vi "动态时值缓存指数压缩.vi"(6 "新数据":cluster{"时间":timestamp, "数值":dbl}, 11 "缓存数据":T1) -> (3 "缓存数据 o":T1)   [LabVIEW 2017, in "时值缓存压缩模块.lvlib"]
doc: "注意：\n缓存容量要在输入数据中设好，默认容量 300 点。"
panel:
  out "Error Out":errorcluster caption="错误输出"
  in  "Error In":errorcluster caption="错误输入"
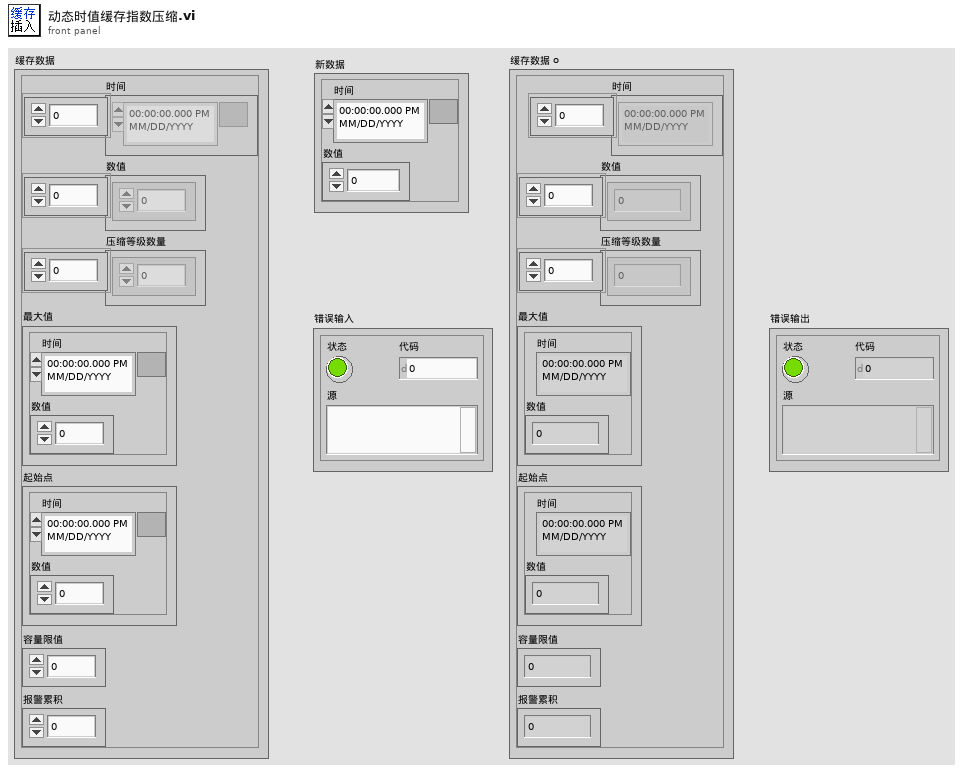
[diagram p1: front panel]
types:
  T1 = typedef "时值缓存压缩模块.lvlib/缓存数据.ctl" = cluster{"时间":timestamp[], "数值":dbl[], "压缩等级数量":i32[], "最大值":cluster{"时间":timestamp, "数值":dbl}, "起始点":cluster{"时间":timestamp, "数值":dbl}, "容量限值":i32, "报警累积":dbl}
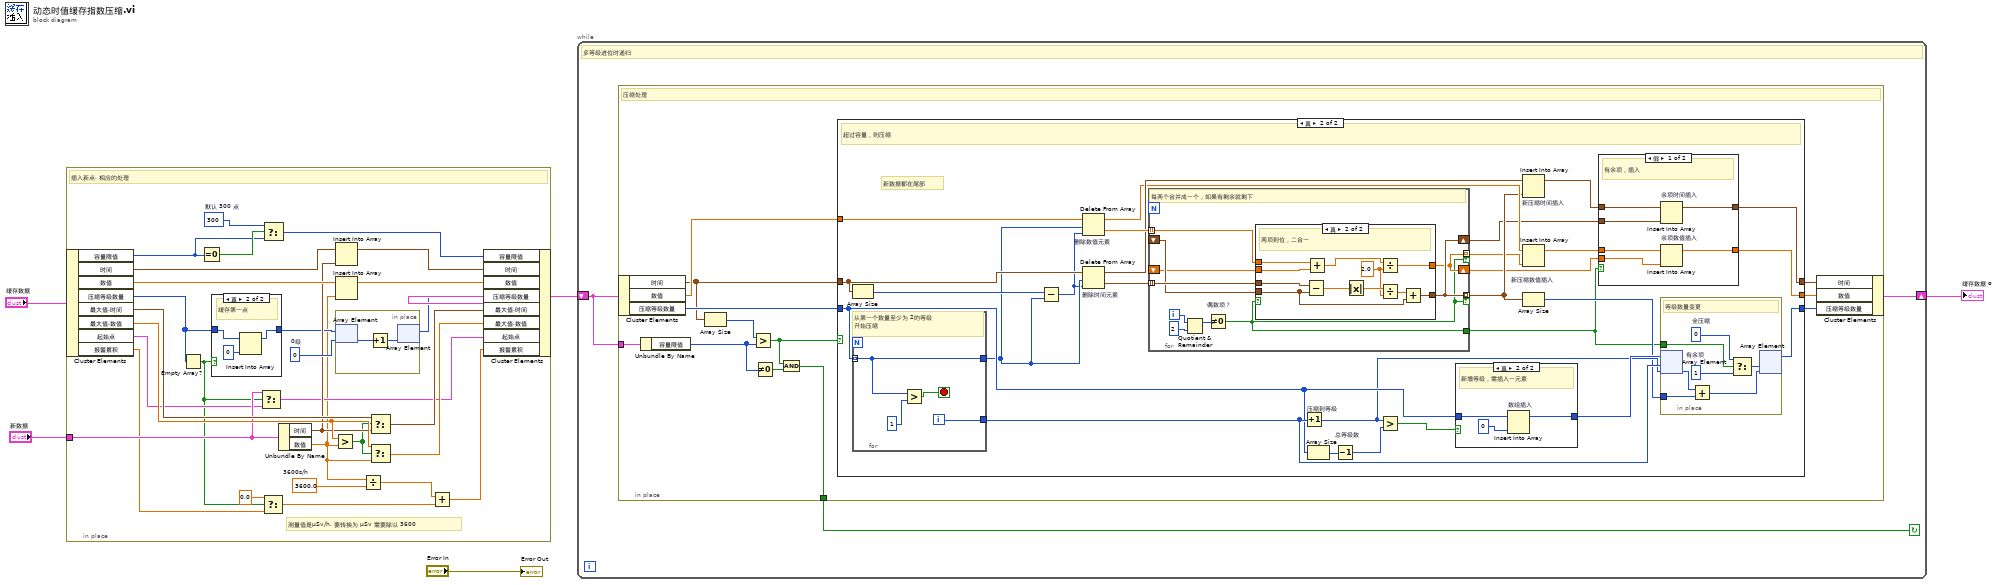
[diagram p0: block diagram]
diagram:
  n1 = in-place {
    in-place-border: "新数据" -> [w20]
    w6 = 3600.0  # 3600s/h
    w16 = 300  # 默认 300 点
    w32 = 0  # 0级
    # "测量值是μSv/h, 要转换为 μSv 需要除以 3600"
    # "插入新点, 相应的处理"
    n2 = in-place-cluster #1("缓存数据") -> ("容量限值"=w15:i32, "时间"=w34:timestamp[], "数值"=w33:dbl[], "压缩等级数量"=w22:i32[], "最大值.时间"=w28:timestamp, "最大值.数值"=w27:dbl, "起始点"=w19:cluster{"时间":timestamp, "数值":dbl}, "报警累积"=w10:dbl)
    n3 = Empty Array?(array=w22) -> (empty?=w12:bool)
    n4 = Equal To 0?(x=w15) -> (x = 0?=w17:bool)
    n5 = case shown="真" w12 {
      tunnel: w22 -> [w35 w38]
      tunnel: [w35 w36] -> w21
      frame False {
        # "不是第一点"
      }
      frame True {
        # "缓存第一点"
        n6 = Insert Into Array(array=w38, new element=0 ("新元素/子数组")) -> (w36:i32[])  [unwired: 1 in]
      }
    }
    n7 = Select(t=w20, s=w12, f=w19) -> (s? t:f=w18:cluster{"时间":timestamp, "数值":dbl})
    n8 = Select(t=0.0, s=w12, f=w10) -> (s? t:f=w9:dbl)
    n9 = Select(t=w16, s=w17, f=w15) -> (s? t:f=w14:i32)
    n10 = Unbundle By Name(w20) -> ("时间"=w26:timestamp, "数值"=w13:dbl)
    n11 = Greater?(x=w27, y=w13) -> (0:w25:bool)
    n12 = Insert Into Array(array=w34, new element=w26) -> (w29:timestamp[])  [unwired: 1 in]
    n13 = Insert Into Array(array=w33, new element=w13) -> (w30:dbl[])  [unwired: 1 in]
    n14 = in-place {
      n15 = in-place-array #2(w21, w32) -> (w40:i32)
      n16 = Increment(x=w40) -> (x+1=w39:i32)
      n17 = in-place-array #2(w39) -> (w31:i32[])  [unwired: 1 out]
    }
    n18 = Divide(x=w13, y=w6) -> (x/y=w7:dbl)
    n19 = Select(t=w28, s=w25, f=w26) -> (s? t:f=w24:timestamp)
    n20 = Select(t=w27, s=w25, f=w13) -> (s? t:f=w23:dbl)
    n21 = Add(x=w7, y=w9) -> (x+y=w8:dbl)
    n22 = in-place-cluster #1("容量限值"=w14, "时间"=w29, "数值"=w30, "压缩等级数量"=w31, "最大值.时间"=w24, "最大值.数值"=w23, "起始点"=w18, "报警累积"=w8) -> (w3:T1)
  }
  n23 = while {
    shift-right: [w42] -> w2
    shift-left: w3 -> [w43]
    stop <- w41 continue-if-true
    # "多等级进位时递归"
    n24 = in-place {
      in-place-border: w43 -> [w48]
      in-place-border: [w45] -> w41
      # "压缩处理"
      n25 = in-place-cluster #3(w43) -> ("时间"=w52:timestamp[], "数值"=w55:dbl[], "压缩等级数量"=w54:i32[])
      n26 = Unbundle By Name(w48) -> ("容量限值"=w46:i32)
      n27 = Array Size(array=w52) -> (size(s)=w53:i32)
      n28 = Greater?(x=w53, y=w46) -> (0:w47:bool)
      n29 = Not Equal To 0?(x=w46) -> (x != 0?=w44:bool)
      n30 = And(x=w47, y=w44) -> (x .and. y?=w45:bool)
      n31 = case shown="真" w47 {
        tunnel: w55 -> [w57 w73]
        tunnel: w52 -> [w58 w74]
        tunnel: [w58 w61] -> w51
        tunnel: [w57 w60] -> w50
        tunnel: [w56 w76] -> w49
        tunnel: w54 -> [w56 w80]
        frame False {
          # "没超过容量就通过"
        }
        frame True {
          # "新数据都在尾部"
          # "超过容量，则压缩"
          n32 = Array Size(array=w74) -> (size(s)=w85:i32)
          n33 = for {
            tunnel: w80 -> [w130] mode=indexing
            tunnel: [w131] -> w83
            tunnel: [w130] -> w72
            i -> [w131]
            stop <- w128 stop-if-true
            # "从第一个数量至少为 2的等级\n开始压缩"
            n34 = Greater?(x=w130, y=1) -> (0:w128:bool)
          }
          n35 = Subtract(x=w85, y=w72) -> (x-y=w71:i32)
          n36 = Delete From Array "删除数值元素"(array=w73, length=w72, index=w71) -> (deleted portion=w70:dbl[], array with subset deleted=w68:dbl[])
          n37 = Delete From Array "删除时间元素"(array=w74, length=w72, index=w71) -> (deleted portion=w75:timestamp[], array with subset deleted=w69:timestamp[])
          n38 = for {
            tunnel: w75 -> [w111] mode=indexing
            tunnel: w70 -> [w110] mode=indexing
            shift-right: [w107] -> w63
            shift-left: _ -> [w109]
            shift-right: [w106] -> w62
            shift-left: _ -> [w108]
            tunnel: [w107] -> w67 mode=indexing if=w105
            tunnel: [w106] -> w66 mode=indexing if=w105
            tunnel: [w105] -> w59
            i -> [w114]
            # "每两个合并成一个，如果有剩余就剩下"
            n39 = Quotient & Remainder(x=w114, y=2) -> (x-y*floor(x/y)=w112:i32)  [unwired: 1 out]
            n40 = Not Equal To 0? "偶数项？"(x=w112) -> (x != 0?=w105:bool)
            n41 = case shown="真" w105 {
              tunnel: [w116 w122] -> w107
              tunnel: w111 -> [w116 w127]
              tunnel: [w115 w118] -> w106
              tunnel: w110 -> [w115 w121]
              tunnel: w109 -> [_ w123]
              tunnel: w108 -> [_ w120]
              frame False {
                # "单独一项，传到下一帧"
              }
              frame True {
                w117 = 2.0 ("y")
                # "两项到位，二合一"
                n42 = Subtract(x=w127, y=w123) -> (x-y=w126:dbl)
                n43 = Add(x=w121, y=w120) -> (x+y=w119:dbl)
                n44 = Absolute Value(x=w126) -> (abs(x)=w125:dbl)
                n45 = Divide(x=w119, y=w117) -> (x/y=w118:dbl)
                n46 = Divide(x=w125, y=w117) -> (x/y=w124:dbl)
                n47 = Add(x=w124, y=w123) -> (x+y=w122:timestamp)
              }
            }
          }
          n48 = Increment "压缩到等级"(x=w83) -> (x+1=w78:i32)
          n49 = Array Size(array=w80) -> (size(s)=w84:i32)
          n50 = Decrement "总等级数"(x=w84) -> (x-1=w82:i32)
          n51 = Greater?(x=w78, y=w82) -> (0:w81:bool)
          n52 = case shown="真" w81 {
            tunnel: w80 -> [w94 w97]
            tunnel: [w94 w95] -> w79
            frame False {
              # "未新增等级，则通过"
            }
            frame True {
              # "新增等级，需插入一元素"
              n53 = Insert Into Array "数组插入"(array=w97, new element=0 ("新元素/子数组")) -> (w95:i32[])  [unwired: 1 in]
            }
          }
          n54 = Insert Into Array "新压缩时间插入"(array=w69, new element=w67) -> (w65:timestamp[])  [unwired: 1 in]
          n55 = Insert Into Array "新压缩数值插入"(array=w68, new element=w66) -> (w64:dbl[])  [unwired: 1 in]
          n56 = Array Size(array=w67) -> (size(s)=w77:i32)
          n57 = case shown="假" w59 {
            tunnel: w65 -> [w91 w93]
            tunnel: w64 -> [w90 w92]
            tunnel: w63 -> [w89 _]
            tunnel: w62 -> [w88 _]
            tunnel: [w87 w92] -> w60
            tunnel: [w86 w93] -> w61
            frame False {
              # "有余项，插入"
              n58 = Insert Into Array "余项时间插入"(array=w91, new element=w89) -> (w86:timestamp[])  [unwired: 1 in]
              n59 = Insert Into Array "余项数值插入"(array=w90, new element=w88) -> (w87:dbl[])  [unwired: 1 in]
            }
            frame True {
              # "全压缩，通过"
            }
          }
          n60 = in-place {
            in-place-border: w59 -> [w103]
            in-place-border: w77 -> [w98]
            w102 = 1  # 有余项
            w104 = 0  # 全压缩
            # "等级数量变更"
            n61 = in-place-array #4(w79, w83, w78) -> (w101:i32)  [unwired: 1 out]
            n62 = Add(x=w101, y=w98) -> (x+y=w99:i32)
            n63 = Select(t=w104, s=w103, f=w102) -> (s? t:f=w100:i32)
            n64 = in-place-array #4(w100, w99) -> (w76:i32[])  [unwired: 2 out]
          }
        }
      }
      n65 = in-place-cluster #3("时间"=w51, "数值"=w50, "压缩等级数量"=w49) -> (w42:T1)
    }
  }
  "缓存数据 o" <- w2
  "Error Out" <- "Error In"
